vi "Apply Settings.vi"(8 "error in (no error)":errorcluster, 11 "VacuumLine in":refnum<class "VacuumLine.lvclass">) -> (0 "error out":errorcluster, 3 "VacuumLine out":refnum<class "VacuumLine.lvclass">)   [LabVIEW 2016, in "Hardware.lvlib" / "VacuumLine.lvlib" / "VacuumLine.lvclass"]
uses:
  <userlib>/Common Components/Hardware/Abstract System/VacuumLine/VacuumLine/VacuumLine.lvclass
  <userlib>/Common Components/Hardware/Motor/Motor/Motor.lvclass
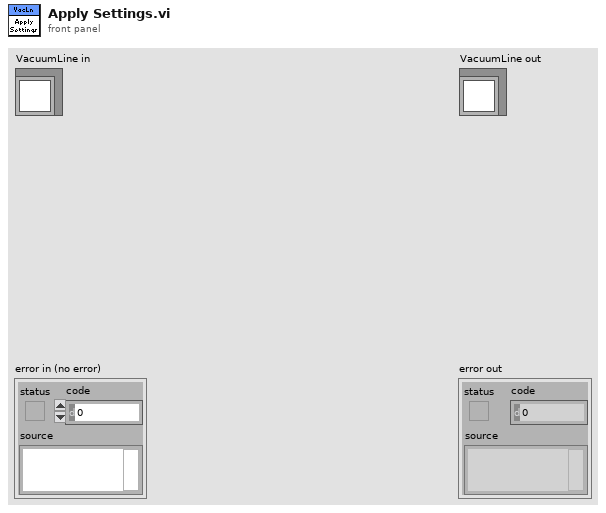
[diagram p1: front panel]
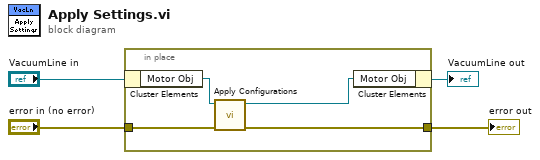
[diagram p0: block diagram]
diagram:
  n1 = in-place {
    in-place-border: "error in (no error)" -> [w6]
    in-place-border: [w5] -> w1
    n2 = in-place-cluster #1("VacuumLine in") -> ("Motor Obj"=w8:refnum<class "Motor.lvclass">)
    n3 = call-dynamic "Apply Configurations.vi"("error in (no error)"=w6, "Motor in"=w8) -> ("error out"=w5:errorcluster, "Motor out"=w7:refnum<class "Motor.lvclass">)  [unwired: 8 in]
    n4 = in-place-cluster #1("Motor Obj"=w7) -> (→"VacuumLine out":refnum<class "VacuumLine.lvclass">)
  }
  "error out" <- w1
